vi "grow_pops.vi"(0 "rho+ array":dbl[](array[numeric]), 1 "Microwave power":dbl, 2 "Zero Level Power":dbl, 3 "Decay rate":dbl, 5 "rho0 array":dbl[](array[numeric]), 7 "Zero Ensemble Condition":dbl[](array[numeric]), 9 "rho- array":dbl[](array[numeric]), 11 "Sat pol":dbl, 12 "I array":dbl[](array[numeric]), 13 "Zero Ensemble Array":dbl[](array[numeric])) -> (4 "rho+ array out":dbl[](array[numeric]), 6 "rho0 array out":dbl[](array[numeric]), 8 "rho0 decay out":dbl[](array[numeric]), 10 "rho- array out":dbl[](array[numeric]), 15 "Zero Ensemble Out":dbl[](array[numeric]))   [LabVIEW 2018]
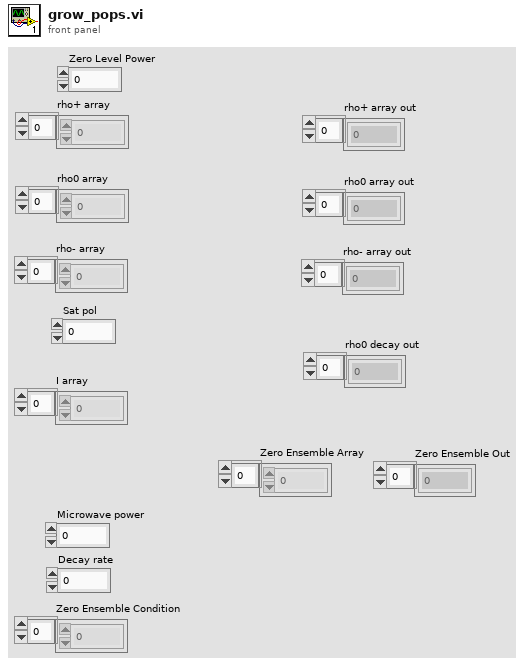
[diagram p1: front panel]
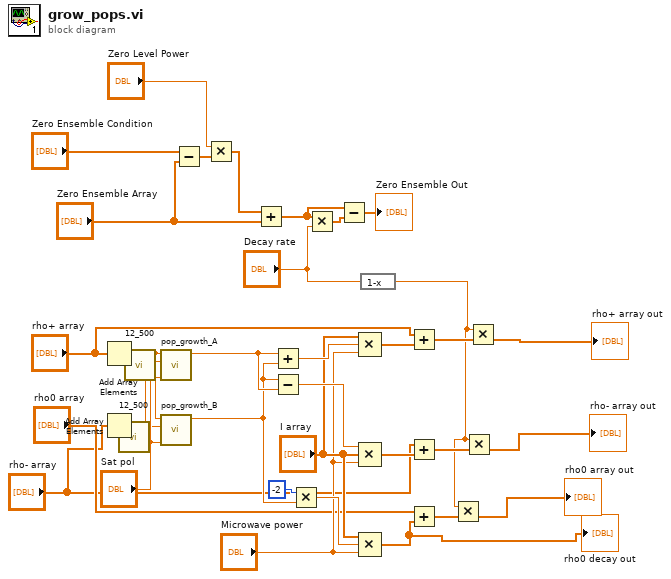
[diagram p0: block diagram]
diagram:
  n1 = Add Array Elements(numeric array="rho+ array") -> (sum=w25:dbl)
  n2 = Add Array Elements(numeric array="rho- array") -> (sum=w26:dbl)
  n3 = call "12_500.vi"("Numeric in"=w26) -> ("Numeric out"=w2:dbl)  [unwired: 10 in]
  n4 = call "12_500.vi"("Numeric in"=w25) -> ("Numeric out"=w1:dbl)  [unwired: 10 in]
  n5 = call "pop_growth_A.vi"("sat pol in"="Sat pol", "rho - val in"=w2, "rho+ val in"=w1) -> ("Growth val out"=w24:dbl)  [unwired: 8 in]
  n6 = call "pop_growth_B.vi"("sat pol in"="Sat pol", "rho - val in"=w2, "rho + val in"=w1) -> ("Growth val out"=w23:dbl)  [unwired: 8 in]
  n7 = Subtract(x="Zero Ensemble Condition", y="Zero Ensemble Array") -> (x-y=w33:dbl[])
  n8 = Multiply(x="Zero Level Power", y=w33) -> (x*y=w32:dbl[])
  n9 = Add(x=w32, y="Zero Ensemble Array") -> (x+y=w29:dbl[])
  n10 = Add(x=w24, y=w23) -> (x+y=w21:dbl)
  n11 = Subtract(x=w23, y=w24) -> (x-y=w20:dbl)
  n12 = Multiply(x=-2, y=w23) -> (x*y=w19:dbl)
  n13 = Multiply(x=w29, y="Decay rate") -> (x*y=w30:dbl[])
  n14 = Subtract(x=w29, y=w30) -> (x-y=→"Zero Ensemble Out":dbl[])
  n15 = Compound Arithmetic op=MULTIPLY("I array", w21, "Microwave power") -> (w16:dbl[])
  n16 = Compound Arithmetic op=MULTIPLY(w20, "I array", "Microwave power") -> (w15:dbl[])
  n17 = Compound Arithmetic op=MULTIPLY("I array", w19, "Microwave power") -> (w9:dbl[])
  "rho0 decay out" <- w9
  n18 = expression code="1-x"("Decay rate") -> (w4:dbl)
  n19 = Add(x="rho+ array", y=w16) -> (x+y=w10:dbl[])
  n20 = Add(x="rho- array", y=w15) -> (x+y=w14:dbl[])
  n21 = Add(x="rho0 array", y=w9) -> (x+y=w12:dbl[])
  n22 = Multiply(x=w4, y=w12) -> (x*y=→"rho0 array out":dbl[])
  n23 = Multiply(x=w4, y=w14) -> (x*y=→"rho- array out":dbl[])
  n24 = Multiply(x=w4, y=w10) -> (x*y=→"rho+ array out":dbl[])
